vi "Extract Top Number.vi"() -> ()   [LabVIEW 2015]
uses:
  <vilib>/Utility/file.llb/Read Delimited Spreadsheet (string).vi
  <vilib>/Utility/file.llb/Write Delimited Spreadsheet (string).vi
panel:
  out "filenames":string[](array[string])
  out "String":string
  in  "file path (dialog if empty)":path=path "J:/Sort/TV/path.txt"
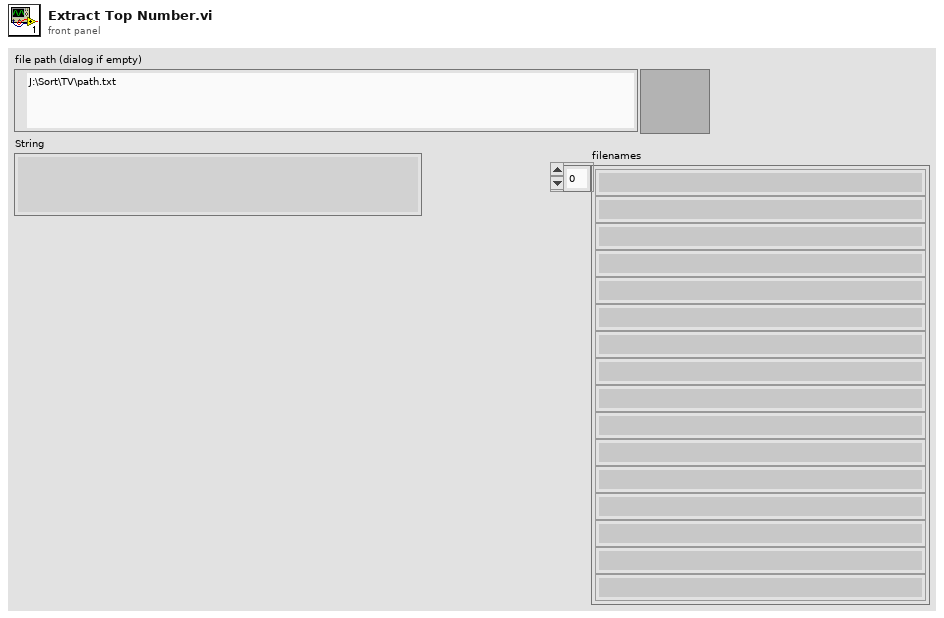
[diagram p1: front panel]
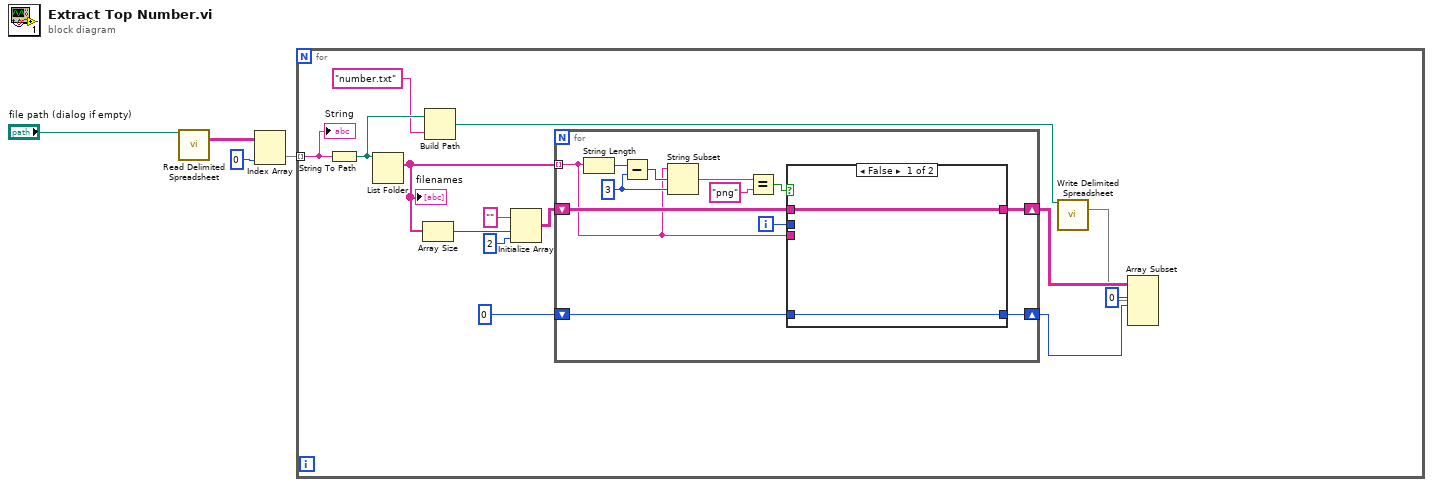
[diagram p0: block diagram]
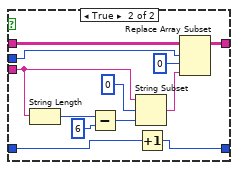
[diagram p2: hidden frame]
diagram:
  n1 = call-poly <vilib>:"Read Delimited Spreadsheet.vi"("file path (dialog if empty)"="file path (dialog if empty)") -> ("all rows"=w3:string[][])  [unwired: 9 in, 5 out]
  n2 = Index Array(array=w3, index (col)=0 ("disabled index (col)")) -> (element=w1:string[])  [unwired: 1 in]
  n3 = for {
    tunnel: w1 -> [w18] mode=indexing
    n4 = String To Path(string=w18) -> (path=w17:path)
    n5 = List Folder(path=w17) -> (filenames=w14:string[])  [unwired: 3 in, 3 out]
    "filenames" <- w14
    n6 = Array Size(array=w14) -> (size(s)=w12:i32)
    n7 = Build Path(base path=w17, name or relative path="number.txt") -> (appended path=w15:path)
    n8 = Initialize Array("", w12, 2 ("dimension size")) -> (w10:string[][])
    n9 = for {
      tunnel: w14 -> [w22] mode=indexing
      shift-right: [w21] -> w8
      shift-left: w10 -> [w24]
      shift-right: [w19] -> w5
      shift-left: 0 ("offset (0)") -> [w20]
      i -> [w23]
      w28 = 3 ("y")
      n10 = String Length(string=w22) -> (length=w30:i32)
      n11 = Subtract(x=w30, y=w28) -> (x-y=w29:i32)
      n12 = String Subset(string=w22, offset (0)=w29, length (rest)=w28) -> (substring=w27:string)
      n13 = Equal?(x=w27, y="png") -> (x = y?=w25:bool)
      n14 = case shown="False" w25 {
        tunnel: w24 -> [w32 w40]
        tunnel: w23 -> [_ w39]
        tunnel: w22 -> [_ w37]
        tunnel: [w32 w35] -> w21
        tunnel: w20 -> [w31 w34]
        tunnel: [w31 w33] -> w19
        frame False {
        }
        frame True {
          n15 = String Length(string=w37) -> (length=w42:i32)
          n16 = Subtract(x=w42, y=6) -> (x-y=w44:i32)
          n17 = String Subset(string=w37, offset (0)=0, length (rest)=w44) -> (substring=w36:string)
          n18 = Increment(x=w34) -> (x+1=w33:i32)
          n19 = Replace Array Subset(array=w40, new element=w36, index (row)=w39, index (col)=0 ("disabled index (col)")) -> (w35:string[][])
        }
      }
    }
    n20 = Array Subset(array=w8, index (row)=0 ("index"), length (row)=w5) -> (w6:string[][])  [unwired: 2 in]
    n21 = call-poly <vilib>:"Write Delimited Spreadsheet.vi"("file path (dialog if empty)"=w15, "2D data"=w6) -> ()  [unwired: 12 in, 2 out]
    "String" <- w18
  }
